vi "FPGA Main Daimler Slow.vi"() -> ()   [LabVIEW 2018]
doc: "This VI reads all analogue data channels available at the fastest rate supported by the respective hardware and updates a memory address for when each measurement is available.\n\nAt a rate defined by the fastest module (NI 9237 - default of 12.5kHz) this memory is read, combined with the measurements from the 9237 module and written to the FIFO for communication to the RT machine.\n\nThe NI 9237 modeul therefore defines the nominal sampling rate of the system (with slower channels over-sampled).\n\nA time channel (in uSec) is provided with 0 referenced from the first acquisition of the NI 9237 module"
uses:
  <vilib>/LabVIEW Targets/FPGA/cRIO/shared/nicrio_ModuleControls/nicrio_cRIO-9237_DataRatesRing.ctl
  <vilib>/rvi/Emulation/niFpgaGetClockAttributes.vi
  <vilib>/rvi/Emulation/niFpgaSctlEmulationGetInTimedLoop.vi
  <vilib>/rvi/Emulation/niFpgaEmulationReportErrorSimple.vi
  <vilib>/rvi/Emulation/niFpgaProcessEmulError.vi
  <vilib>/rvi/eio/common/nirviEmuTemplatePropertySet_noerrors.vi
  <vilib>/rvi/eio/common/nirviEmuTemplateMethod_errors.vi
  <vilib>/rvi/interface/RandomDataEmulation/niFpgaRandomDataHandleErrors.vi
  <vilib>/rvi/Memory/Memory_Emulation/nirvimemoryFastEmulation.vi
  <vilib>/rvi/Memory/Memory_Emulation/nirvimemoryEmulation.vi
  <vilib>/rvi/Emulation/niFpgaEmulationIsFPGAContextNoSignature.vi
  <vilib>/rvi/DataTransferAndStorage/Container/Common/niFpgaContainerGetUniqueNameForEmu.vi
  <vilib>/rvi/errors/nirviReportUnexpectedCaseInternalError (U32).vi
  <vilib>/rvi/Emulation/niFpgaCriticalErrorInLSC.vi
  <vilib>/eio/EIOPropertyNode/EIOPropertyNode.xnode
  <vilib>/LabVIEW Targets/FPGA/cRIO/shared/nicrio_ModuleControls/nicrio_cRIO-9239_DataRatesRing.ctl
  <vilib>/eio/EIONode/EIONode.xnode
  <vilib>/rvi/DataTransferAndStorage/Container/XNode/niFpgaContainer.xnode
  <vilib>/rvi/interface/RandomDataEmulation/nirviRandomDataFpgaReadWriteTemplate.vi
  <vilib>/eio/EIOMethodNode/EIOMethodNode.xnode
  <vilib>/rvi/eio/common/nirviEmuTemplatePropertyGet_errors.vi
  <vilib>/rvi/eio/common/nirviEmuTemplatePropertyGet_noerrors.vi
  <vilib>/rvi/eio/common/nirviEmuTemplatePropertySet_errors.vi
panel:
  in  "active_channels":bool[](array[boolean])=[FALSE, FALSE, FALSE, FALSE, FALSE, FALSE, FALSE, FALSE, FALSE, FALSE, FALSE, FALSE, FALSE, FALSE, FALSE, FALSE, FALSE, FALSE, FALSE, FALSE, FALSE, FALSE, FALSE, FALSE, FALSE, FALSE, FALSE, FALSE, FALSE, FALSE, FALSE, FALSE, FALSE, FALSE, FALSE, FALSE, FALSE, FALSE, FALSE, FALSE, FALSE, FALSE, FALSE, FALSE, FALSE, FALSE, FALSE, FALSE, FALSE, FALSE, FALSE, FALSE, FALSE, FALSE, FALSE, FALSE, FALSE, FALSE, FALSE, FALSE, FALSE, FALSE, FALSE]
  in  "Data Rate":T1=1 items=["50.000 kS/s (NI 9237)"=1, "25.000 kS/s (NI 9237)"=2, "16.667 kS/s (NI 9237)"=3, "12.500 kS/s (NI 9237)"=4, "10.000 kS/s (NI 9237)"=5, "8.333 kS/s (NI 9237)"=6, "7.143 kS/s (NI 9237)"=7, "6.250 kS/s (NI 9237)"=8, "5.556 kS/s (NI 9237)"=9, "5.000 kS/s (NI 9237)"=10, "4.545 kS/s (NI 9237)"=11, "4.167 kS/s (NI 9237)"=12, "3.846 kS/s (NI 9237)"=13, "3.571 kS/s (NI 9237)"=14, "3.333 kS/s (NI 9237)"=15, "3.125 kS/s (NI 9237)"=16, "2.941 kS/s (NI 9237)"=17, "2.778 kS/s (NI 9237)"=18, "2.632 kS/s (NI 9237)"=19, "2.500 kS/s (NI 9237)"=20, "2.381 kS/s (NI 9237)"=21, "2.273 kS/s (NI 9237)"=22, "2.174 kS/s (NI 9237)"=23, "2.083 kS/s (NI 9237)"=24, "2.000 kS/s (NI 9237)"=25, "1.923 kS/s (NI 9237)"=26, "1.852 kS/s (NI 9237)"=27, "1.786 kS/s (NI 9237)"=28, "1.724 kS/s (NI 9237)"=29, "1.667 kS/s (NI 9237)"=30, "1.613 kS/s (NI 9237)"=31]
  out "Total channel count":u32=61
  out "timestamp":u32
  out "FIFO full counter":i32
  in  "Voltage Out":fxp<+/-,20,5>[](array[numeric])=[0.0, 0.0, 0.0, 0.0]
  in  "Update Outputs":bool
  in  "Mod 8":bool[](array[boolean])=[FALSE, FALSE, FALSE, FALSE, FALSE, FALSE, FALSE, FALSE]
  in  "Stop acquire":bool
  # "Torque Measurement"
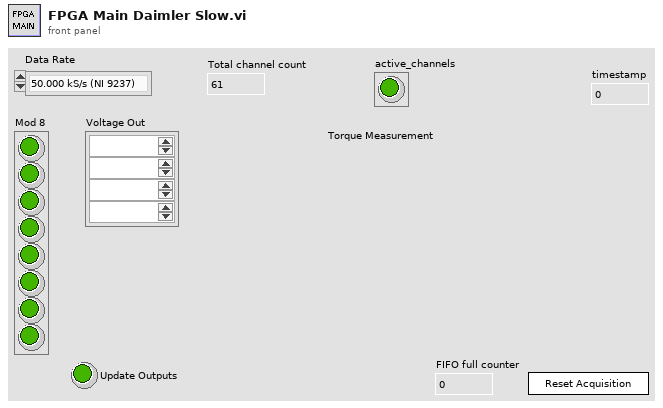
[diagram p1: front panel]
types:
  T1 = typedef "nicrio_cRIO-9237_DataRatesRing.ctl" = u8
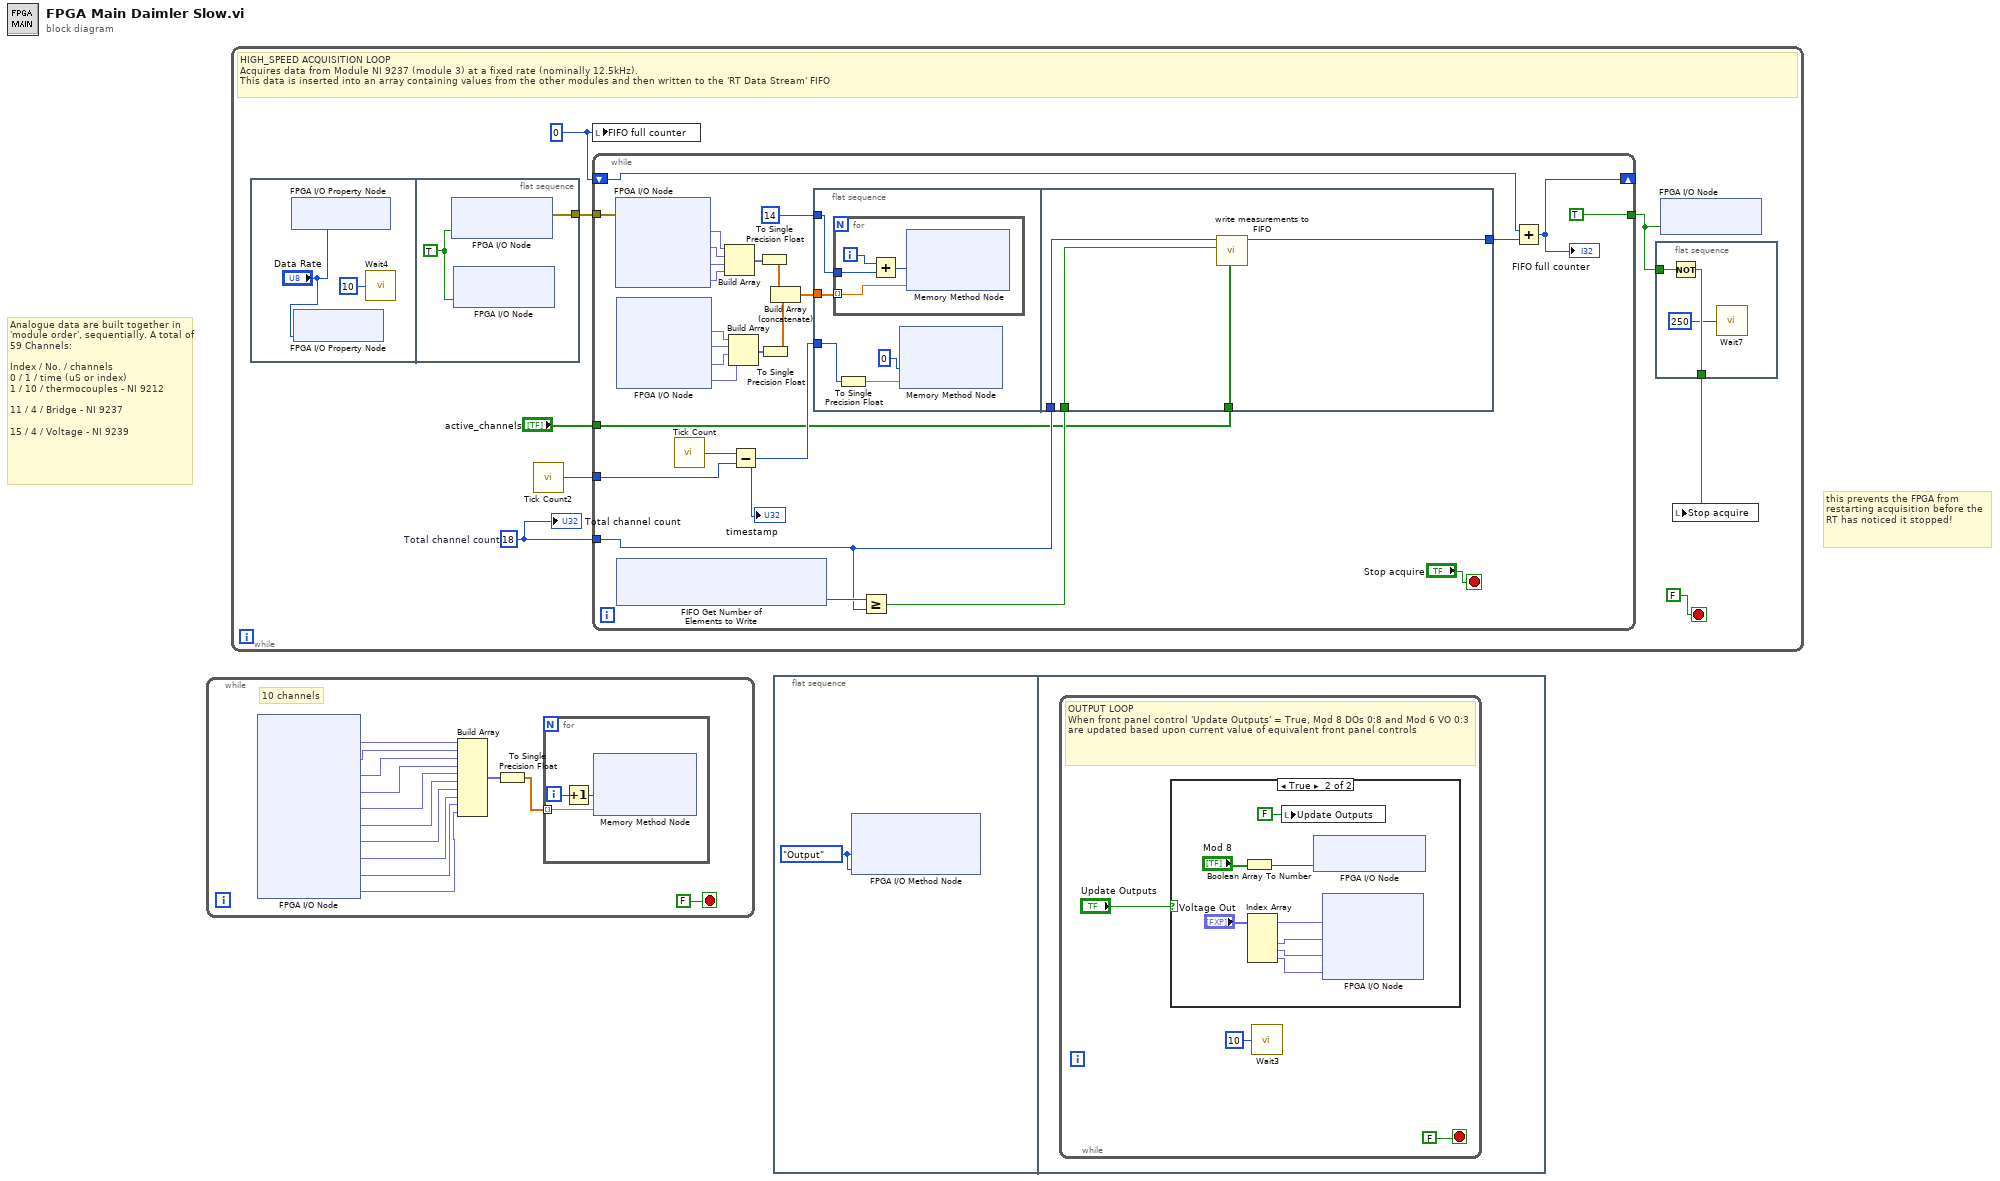
[diagram p0: block diagram]
diagram:
  # "this prevents the FPGA from restarting acquisition before the RT has noticed it stopped!"
  # "Analogue data are built together in 'module order', sequentially. A total of 59 Channels:\n\nIndex / No. / channels\n0 / 1 / time (uS or index)\n1 / 10 / thermocouples - NI 9212\n\n11 / 4 / Bridge - NI 9237\n\n15 / 4 / Voltage - NI 9239"
  n1 = while {
    stop <- FALSE stop-if-true
    # "10 channels"
    n2 = xnode "FPGA I/O Node"() -> ("Mod1/TC0"=w13:fxp<+/-,24,-2>, "Mod1/TC1"=w12:fxp<+/-,24,-2>, "Mod1/TC2"=w11:fxp<+/-,24,-2>, "Mod1/TC3"=w10:fxp<+/-,24,-2>, "Mod1/TC4"=w9:fxp<+/-,24,-2>, "Mod1/TC5"=w8:fxp<+/-,24,-2>, "Mod1/TC6"=w7:fxp<+/-,24,-2>, "Mod1/TC7"=w6:fxp<+/-,24,-2>, "Mod1/CJC0"=w3:fxp<+/-,24,-2>, "Mod1/CJC1"=w2:fxp<+/-,24,-2>)  [unwired: 10 in, 10 out]
    n3 = Build Array(w13, w12, w11, w10, w9, w8, w7, w6, w3, w2) -> (w5:fxp<+/-,24,-2>[])
    n4 = To Single Precision Float(number=w5) -> (single precision float=w4:sgl[])
    n5 = for {
      tunnel: w4 -> [w16] mode=indexing
      i -> [w15]
      n6 = Increment(x=w15) -> (x+1=w14:i32)
      n7 = xnode ("Memory Method Node")("Address"=w14, "Data"=w16) -> ()  [unwired: 1 in, 1 out]
    }
  }
  n8 = while {
    stop <- FALSE stop-if-true
    w19 = 0 ("FIFO full counter")
    w22 = u32 18  # Total channel count
    # "HIGH_SPEED ACQUISITION LOOP\nAcquires data from Module NI 9237 (module 3) at a fixed rate (nominally 12.5kHz).\nThis data is inserted into an array containing values from the other modules and then written to the 'RT Data Stream' FIFO"
    n9 = flat-sequence {
      tunnel: [w31] -> w23
      frame #0 {
        n10 = xnode "FPGA I/O Property Node"("Data Rate"="Data Rate") -> ()  [unwired: 1 in, 1 out]
        n11 = xnode "FPGA I/O Property Node"("Data Rate"="Data Rate") -> ()  [unwired: 1 in, 1 out]
        n12 = call "Wait4"("Count(mSec)"=u16 10) -> ()  [unwired: 1 out]
      }
      frame #1 {
        w30 = TRUE ("Mod3/Start")
        n13 = xnode "FPGA I/O Node"("Mod3/Start"=w30) -> ("error out"=w31:errorcluster)  [unwired: 2 in, 1 out]
        n14 = xnode "FPGA I/O Node"("Mod5/Start"=w30) -> ()  [unwired: 2 in, 2 out]
      }
    }
    n15 = call "Tick Count2"() -> ("Tick Count(uSec)"=w24:u32)
    n16 = local write "FIFO full counter"(w19) -> ()
    n17 = while {
      tunnel: [TRUE ("I/O Item")] -> w21
      tunnel: w23 -> [w57]
      tunnel: w22 -> [w42]
      shift-right: [w50] -> _
      shift-left: w19 -> [w48]
      tunnel: w24 -> [w51]
      tunnel: "active_channels" -> [w32]
      stop <- "Stop acquire" stop-if-true
      n18 = xnode "FPGA I/O Node"("error in"=w57) -> ("Mod3/AI0"=w56:fxp<+/-,24,-4>, "Mod3/AI1"=w55:fxp<+/-,24,-4>, "Mod3/AI2"=w54:fxp<+/-,24,-4>, "Mod3/AI3"=w53:fxp<+/-,24,-4>)  [unwired: 4 in, 5 out]
      n19 = xnode "FPGA I/O Node"() -> ("Mod5/AI0"=w39:fxp<+/-,24,5>, "Mod5/AI1"=w38:fxp<+/-,24,5>, "Mod5/AI2"=w37:fxp<+/-,24,5>, "Mod5/AI3"=w36:fxp<+/-,24,5>)  [unwired: 5 in, 5 out]
      n20 = xnode ("FIFO Get Number of Elements to Write")() -> ("Number of Elements to Write"=w44:u32)  [unwired: 1 in, 1 out]
      n21 = call "Tick Count"() -> ("Tick Count(uSec)"=w47:u32)
      n22 = Build Array(w56, w55, w54, w53) -> (w52:fxp<+/-,24,-4>[])
      n23 = Build Array(w39, w38, w37, w36) -> (w35:fxp<+/-,24,5>[])
      n24 = Subtract(x=w47, y=w51) -> (x-y=w40:u32)
      "timestamp" <- w40
      n25 = To Single Precision Float(number=w52) -> (single precision float=w46:sgl[])
      n26 = To Single Precision Float(number=w35) -> (single precision float=w33:sgl[])
      n27 = Build Array (concatenate)(w46, w33) -> (w34:sgl[])
      n28 = flat-sequence {
        tunnel: w34 -> [w63]
        tunnel: 14 ("index") -> [w62]
        tunnel: w40 -> [w60]
        tunnel: w42 -> [w71]
        tunnel: [w70] -> w41
        tunnel: w43 -> [w69]
        tunnel: w32 -> [w68]
        frame #0 {
          n29 = for {
            tunnel: w63 -> [w67] mode=indexing
            tunnel: w62 -> [w66]
            i -> [w64]
            n30 = Add(x=w64, y=w66) -> (x+y=w65:i32)
            n31 = xnode ("Memory Method Node")("Address"=w65, "Data"=w67) -> ()  [unwired: 1 in, 1 out]
          }
          n32 = To Single Precision Float(number=w60) -> (single precision float=w61:sgl)
          n33 = xnode ("Memory Method Node")("Address"=u32 0, "Data"=w61) -> ()  [unwired: 1 in, 1 out]
        }
        frame #1 {
          n34 = call "write measurements to FIFO.vi"("active_channels"=w68, "FIFO space"=w69, "Total channel count"=w71) -> ("FIFO full"=w70:i32)  [unwired: 8 in]
        }
      }
      n35 = Greater Or Equal?(x=w44, y=w42) -> (x >= y?=w43:bool)
      n36 = Add(x=w48, y=w41) -> (x+y=w50:i32)
      "FIFO full counter" <- w50
    }
    n37 = flat-sequence {
      tunnel: w21 -> [w27]
      tunnel: [w26] -> w18
      frame #0 {
        n38 = Not(x=w27) -> (.not. x?=w26:bool)
        n39 = call "Wait7"("Count(mSec)"=u8 250) -> ()  [unwired: 1 out]
      }
    }
    n40 = xnode "FPGA I/O Node"("Mod3/Stop"=w21) -> ()  [unwired: 1 in, 1 out]
    n41 = local write "Stop acquire"(w18) -> ()
    "Total channel count" <- w22
  }
  n42 = flat-sequence {
    frame #0 {
      w72 = enum8{"No Change", "Input", "Output"}."Output" ("DIO 7:4")
      n43 = xnode "FPGA I/O Method Node"("DIO 7:4"=w72, "DIO 3:0"=w72) -> ()  [unwired: 1 in, 1 out]
    }
    frame #1 {
      n44 = while {
        stop <- FALSE stop-if-true
        # "OUTPUT LOOP\nWhen front panel control 'Update Outputs' = True, Mod 8 DOs 0:8 and Mod 6 VO 0:3 are updated based upon current value of equivalent front panel controls"
        n45 = case shown="True" "Update Outputs" {
          frame False {
          }
          frame True {
            n46 = Boolean Array To Number(Boolean array="Mod 8") -> (number=w82:u8)
            n47 = Index Array(array="Voltage Out") -> (element #1=w80:fxp<+/-,20,5>, element #2=w79:fxp<+/-,20,5>, element #3=w77:fxp<+/-,20,5>, element #4=w76:fxp<+/-,20,5>)  [unwired: 4 in]
            n48 = local write "Update Outputs"(FALSE ("Update Outputs")) -> ()
            n49 = xnode "FPGA I/O Node"("Mod8/DIO7:0"=w82) -> ()  [unwired: 1 in, 1 out]
            n50 = xnode "FPGA I/O Node"("Mod6/AO0"=w80, "Mod6/AO1"=w79, "Mod6/AO2"=w77, "Mod6/AO3"=w76) -> ()  [unwired: 4 in, 4 out]
          }
        }
        n51 = call "Wait3"("Count(uSec)"=u16 10 ("Count(Ticks)")) -> ()  [unwired: 1 out]
      }
    }
  }
